vi "Right Click.vi"(7 "object refs":T2, 8 "error in (no error)":errorcluster, 9 "Coords":T1, 10 "Event data":variant, 11 "Multi Column Listbox in":refnum<class "Multi Column Listbox.lvclass">) -> (0 "error out":errorcluster, 3 "Multi Column Listbox out":refnum<class "Multi Column Listbox.lvclass">)   [LabVIEW 2013, in "Table Manager.lvlib" / "Multi Column Listbox.lvclass"]
doc: "Displays the menu options on a Right-Click."
uses:
  Multi Column Listbox.lvclass
  Table Manager/object ref.ctl
  Configuration Editor/Classes/Engine Parent/Engine Parent Editor Node.lvclass
  Configuration Editor/Classes/Module editor node/module editor node.lvclass
  <vilib>/Utility/miscctls.llb/LVPoint32TypeDef.ctl
  Multi Column Listbox.lvclass/Multi Column Listbox.ctl
  <vilib>/NI/Tag Bus/tag/tag descriptor.lvclass
  Table Manager.lvlib
  <vilib>/NI/Tag Bus Module Framework/module configuration/TBM module configuration.lvclass
  Table Manager/Table Manager.lvclass
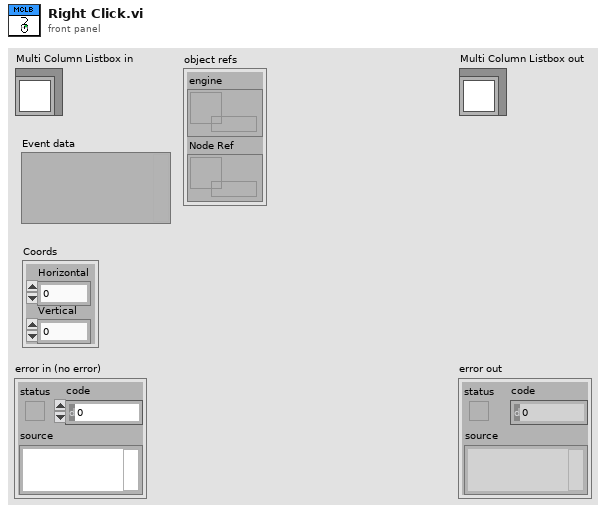
[diagram p1: front panel]
types:
  T1 = typedef "LVPoint32TypeDef.ctl" = cluster{"Horizontal":i32, "Vertical":i32}
  T2 = typedef "Table Manager.lvlib/Table Manager.lvclass/object ref.ctl" = cluster{"engine":refnum<data-value>, "Node Ref":refnum<data-value>}
  T3 = typedef "LVRowAndColumnTypeDef.ctl" = cluster{"Row":i32, "Column":i32}
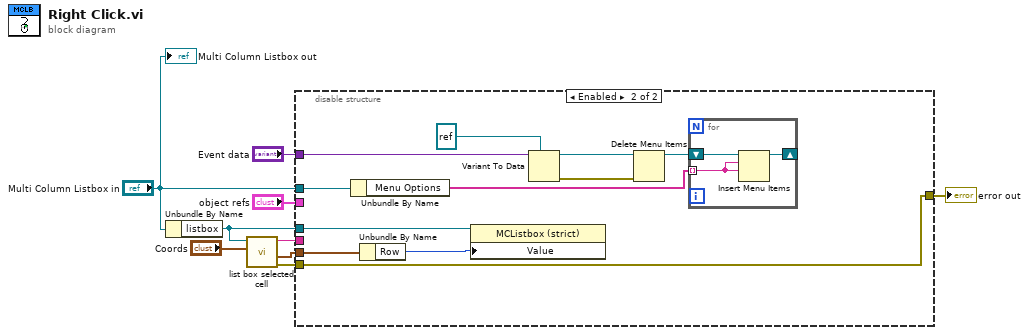
[diagram p0: block diagram]
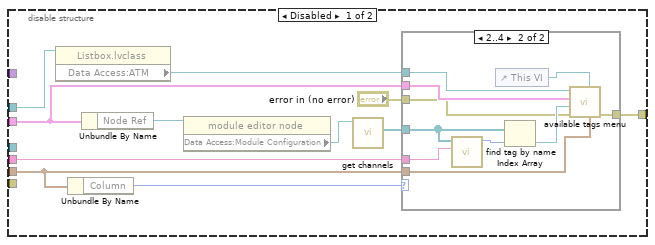
[diagram p2: hidden frame]
diagram:
  n1 = Unbundle By Name("Multi Column Listbox in") -> ("listbox"=w1:refnum<vi>)
  n2 = call "list box selected cell.vi"("Coords"="Coords", "MulticolumnListbox in"=w1) -> ("error out"=w3:errorcluster, "cell position"=w4:T3, "tag select name"=w5:string)  [unwired: 6 in, 1 out]
  n3 = disable-structure shown="Enabled" {
    disable-tunnel: "object refs" -> [w16 _]
    disable-tunnel: [w15 w32] -> w8
    disable-tunnel: "Multi Column Listbox in" -> [w13 w38]
    disable-tunnel: "Event data" -> [_ w42]
    disable-tunnel: w5 -> [w11 _]
    disable-tunnel: w4 -> [w10 w34]
    disable-tunnel: w3 -> [_ w32]
    disable-tunnel: w1 -> [_ w35]
    frame Disabled {
      n4 = property class="Listbox.lvclass"(reference=w13) -> ("Data Access:ATM"=w12:refnum<user-event>)  [unwired: 1 in, 2 out]
      n5 = Unbundle By Name(w10) -> ("Column"=w18:i32)
      n6 = Unbundle By Name(w16) -> ("Node Ref"=w17:refnum<data-value>)
      n7 = property class="module editor node"(reference=w17) -> ("Data Access:Module Configuration"=w20:refnum<class "TBM module configuration.lvclass">)  [unwired: 1 in, 2 out]
      n8 = call-dynamic "get channels.vi"("module configuration in"=w20) -> ("channels"=w19:refnum<class "TBM channel.lvclass">[])  [unwired: 9 in, 1 out]
      n9 = case shown="2..4" w18 {
        tunnel: w19 -> [_ w30]
        tunnel: w11 -> [_ w29]
        tunnel: w12 -> [_ w26]
        tunnel: w16 -> [_ w25]
        tunnel: [w21 w24] -> w15
        tunnel: "error in (no error)" -> [w21 w23]
        tunnel: w10 -> [_ w22]
        frame 0, Default {
        }
        frame 2..4 {
          n10 = call <vilib>:"find tag by name.vi"("name"=w29, "tags in"=w30) -> ("index"=w31:i32)  [unwired: 9 in]
          n11 = control-ref of="This VI"() -> (w28:refnum<vi>)
          n12 = Index Array(array=w30, index=w31) -> (element=w27:refnum<class "TBM channel.lvclass">)
          n13 = call "available tags menu.vi"("Point32"=w22, "parent vi reference"=w28, "error in"=w23, "channel to map to"=w27, "object ref"=w25, "ATM"=w26) -> ("error out"=w24:errorcluster)  [unwired: 5 in]
        }
      }
    }
    frame Enabled {
      n14 = Unbundle By Name(w38) -> ("Menu Options"=w37:string[])
      n15 = Unbundle By Name(w34) -> ("Row"=w33:i32)
      n16 = property class="MCListbox (strict)"(reference=w35, "Value"=w33) -> ()  [unwired: 1 in, 2 out]
      n17 = Variant To Data(type=refnum<k9> refnum ("MenuRef"), Variant=w42) -> (data=w40:refnum<k9>, error out=w39:errorcluster)  [unwired: 1 in]
      n18 = Delete Menu Items(6:w39, 9:w40) -> (3:w36:refnum<k9>)  [unwired: 2 in, 1 out]
      n19 = for {
        tunnel: w37 -> [w45] mode=indexing
        shift-right: [w43] -> _
        shift-left: w36 -> [w44]
        n20 = Insert Menu Items(7:w45, 8:w45, 9:w44) -> (3:w43:refnum<k9>)  [unwired: 3 in, 2 out]
      }
    }
  }
  "error out" <- w8
  "Multi Column Listbox out" <- "Multi Column Listbox in"
